vi "FuncImg-Cleanup.vi"(11 "Event Registration Refnum in":T1) -> ()   [LabVIEW 2017]
uses:
  Typedefs/FuncImg-Events registration ref.ctl
  <vilib>/Utility/miscctls.llb/LVRangeTypeDef.ctl
  Globals/gl_Funct imaging UI.vi
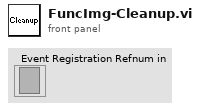
[diagram p1: front panel]
types:
  T1 = typedef "FuncImg-Events registration ref.ctl" = refnum<event-registration>
  T2 = enum32{"Invalid", "Standard", "Closed", "Hidden", "Minimized", "Maximized"}
  T3 = enum32{"invalid app kind", "Development System", "Run Time System", "Student Edition", "Embedded LabVIEW", "Evaluation", "Custom"}
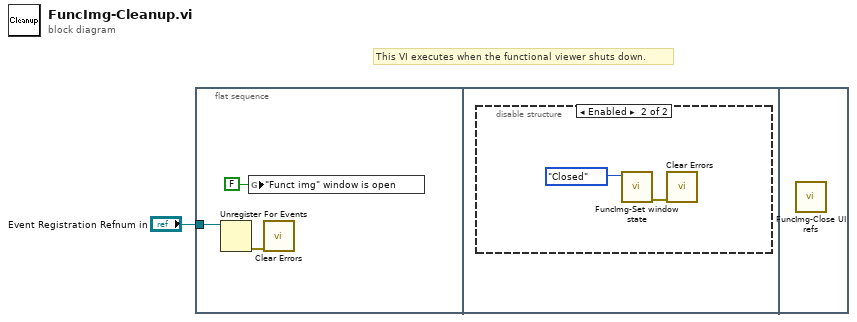
[diagram p0: block diagram]
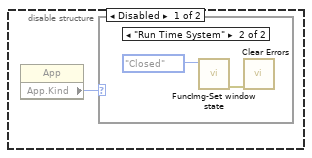
[diagram p2: hidden frame]
diagram:
  # "This VI executes when the functional viewer shuts down."
  n1 = flat-sequence {
    tunnel: "Event Registration Refnum in" -> [w4]
    frame #0 {
      n2 = Unregister For Events(event registration refnum=w4) -> (error out=w2:errorcluster)  [unwired: 1 in]
      n3 = global write "gl_Funct imaging UI.vi" "\"Funct img\" window is open"(FALSE ("\"Funct img\" window is open")) -> ()
      n4 = call <vilib>:"Clear Errors.vi"("error in (no error)"=w2) -> ()  [unwired: 5 in, 2 out]
    }
    frame #1 {
      n5 = disable-structure shown="Enabled" {
        frame Disabled {
          n6 = property class="App"() -> ("App.Kind"=w5:T3)  [unwired: 2 in, 2 out]
          n7 = case shown="\"Run Time System\"" w5 {
            frame Default {
            }
            frame "Run Time System" {
              n8 = call "FuncImg-Set window state.vi"("Front Panel Window:State"=T2."Closed") -> ("error out"=w7:errorcluster)  [unwired: 10 in]
              n9 = call <vilib>:"Clear Errors.vi"("error in (no error)"=w7) -> ()  [unwired: 5 in, 2 out]
            }
          }
        }
        frame Enabled {
          n10 = call "FuncImg-Set window state.vi"("Front Panel Window:State"=T2."Closed") -> ("error out"=w9:errorcluster)  [unwired: 10 in]
          n11 = call <vilib>:"Clear Errors.vi"("error in (no error)"=w9) -> ()  [unwired: 5 in, 2 out]
        }
      }
    }
    frame #2 {
      n12 = call "FuncImg-Close UI refs.vi"() -> ()  [unwired: 12 in]
    }
  }
